vi "x_y_from_graph.vi"(8 "error in (no error)":errorcluster, 11 "graph_reference":refnum<vi>) -> (0 "error out":errorcluster, 2 "y []":dbl[](array[numeric]), 3 "x []":dbl[](array[numeric]))   [LabVIEW 2015, in "lv-calibration.lvlib"]
uses:
  lv-calibration.lvlib
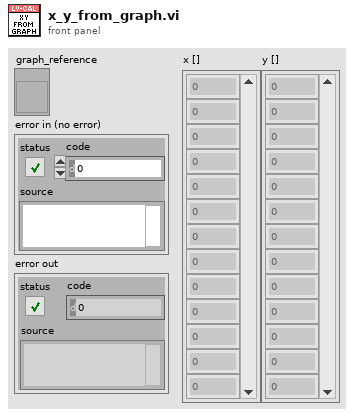
[diagram p1: front panel]
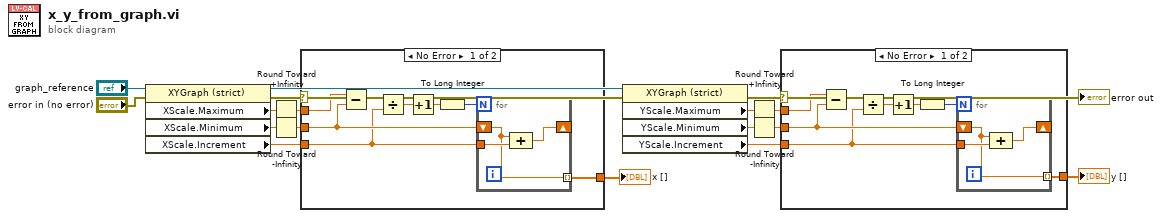
[diagram p0: block diagram]
diagram:
  n1 = property on="Property Node" class="XYGraph (strict)"(reference="graph_reference", error in="error in (no error)") -> (reference out=w13:refnum<vi>, error out=w12:errorcluster, "XScale.Maximum"=w16:dbl, "XScale.Minimum"=w15:dbl, "XScale.Increment"=w14:dbl)
  n2 = Round Toward +Infinity(x=w16) -> (ceil(x): smallest int >= x=w3:dbl)
  n3 = Round Toward -Infinity(1:w15) -> (0:w4:dbl)
  n4 = case shown="No Error" w12 {
    tunnel: w3 -> [w25 _]
    tunnel: w4 -> [w22 _]
    tunnel: w14 -> [w21 _]
    tunnel: [w18 _] -> w11
    frame No Error {
      n5 = Subtract(x=w25, y=w22) -> (x-y=w24:dbl)
      n6 = Divide(x=w24, y=w21) -> (x/y=w23:dbl)
      n7 = Increment(x=w23) -> (x+1=w20:dbl)
      n8 = To Long Integer(number=w20) -> (32bit integer=w19:i32)
      n9 = for {
        N: w19 -> [_]
        tunnel: w21 -> [w28]
        tunnel: [w26] -> w18 mode=indexing
        shift-right: [w27] -> _
        shift-left: w22 -> [w26]
        n10 = Compound Arithmetic op=ADD(w26, w28) -> (w27:dbl)
      }
    }
    frame Error {
    }
  }
  "x []" <- w11
  n11 = property on="Property Node" class="XYGraph (strict)"(reference=w13, error in=w12) -> (error out=w7:errorcluster, "YScale.Maximum"=w10:dbl, "YScale.Minimum"=w9:dbl, "YScale.Increment"=w8:dbl)  [unwired: 1 out]
  "error out" <- w7
  n12 = Round Toward +Infinity(x=w10) -> (ceil(x): smallest int >= x=w1:dbl)
  n13 = Round Toward -Infinity(1:w9) -> (0:w2:dbl)
  n14 = case shown="No Error" w7 {
    tunnel: w1 -> [w36 _]
    tunnel: w2 -> [w33 _]
    tunnel: w8 -> [w32 _]
    tunnel: [w29 _] -> w6
    frame No Error {
      n15 = Subtract(x=w36, y=w33) -> (x-y=w35:dbl)
      n16 = Divide(x=w35, y=w32) -> (x/y=w34:dbl)
      n17 = Increment(x=w34) -> (x+1=w31:dbl)
      n18 = To Long Integer(number=w31) -> (32bit integer=w30:i32)
      n19 = for {
        N: w30 -> [_]
        tunnel: w32 -> [w39]
        tunnel: [w38] -> w29 mode=indexing
        shift-right: [w37] -> _
        shift-left: w33 -> [w38]
        n20 = Compound Arithmetic op=ADD(w38, w39) -> (w37:dbl)
      }
    }
    frame Error {
    }
  }
  "y []" <- w6
